vi "Read Project Path.vi"(8 "error in (no error)":errorcluster, 11 "Run UTF in":refnum<class "Run UTF.lvclass">) -> (0 "error out":errorcluster, 2 "Project Path":path, 3 "Run UTF out":refnum<class "Run UTF.lvclass">)   [LabVIEW 2014, in "Run UTF.lvclass"]
uses:
  Run UTF.lvclass
  Run UTF.lvclass/Run UTF.ctl
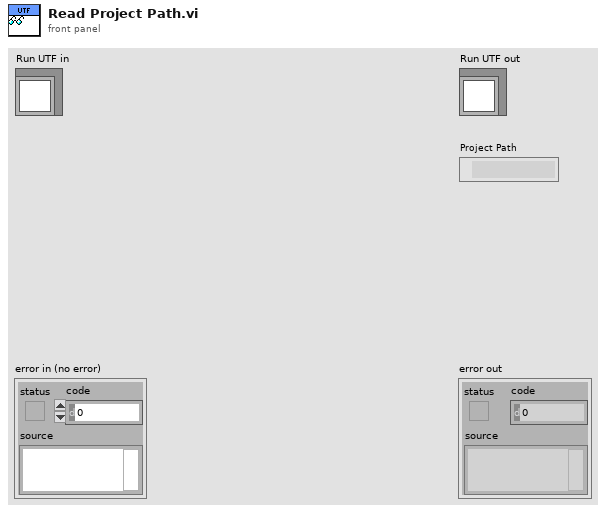
[diagram p1: front panel]
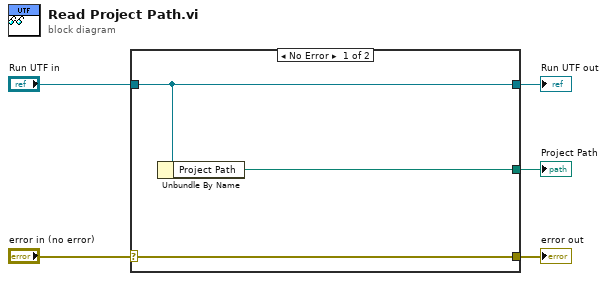
[diagram p0: block diagram]
diagram:
  n1 = case shown="No Error" "error in (no error)" {
    selector: "error in (no error)" -> [w8 w9]
    tunnel: [w8 w9] -> w4
    tunnel: [w7 w10] -> w2
    tunnel: "Run UTF in" -> [w7 w10]
    tunnel: [w6 _] -> w1
    frame No Error {
      n2 = Unbundle By Name(w7) -> ("Project Path"=w6:path)
    }
    frame Error {
    }
  }
  "error out" <- w4
  "Run UTF out" <- w2
  "Project Path" <- w1
